vi "MGI Approximately Equal.vi"(1 "Numeric 2":dbl format="%.2f", 2 "Numeric 1":dbl format="%.2f") -> (0 "approx = ?":bool)   [LabVIEW 2020]
doc: "Check that two floats are within 1% of each other. If either number is zero, then check that they are within Machine Epsilon of each other.\n\nAuthored by David A. Moore\nsupport@mooregoodideas.com\nwww.mooregoodideas.com\n\nCopyright (c) 2010, Moore Good Ideas, Inc.\n\nAll rights reserved.\n\nRedistribution and use in source and binary forms, with or without modification, are permitted provided that the following conditions are met:\n\n * Redistributions of source code must retain the above copyright notice, this list of conditions and the following disclaimer.\n * Redistributions in binary form must reproduce the above copyright notice, this list of conditions and the following disclaimer in the documentation and/or other materials provided with the distribution.\n * Neither the name of Moore Good Ideas, Inc. nor the names of its contributors may be used to endorse or promote products derived from this software without specific prior written permission.\n\nTHIS SOFTWARE IS PROVIDED BY THE COPYRIGHT HOLDERS AND CONTRIBUTORS \"AS IS\" AND ANY EXPRESS OR IMPLIED WARRANTIES, INCLUDING, BUT NOT LIMITED TO, THE IMPLIED WARRANTIES OF MERCHANTABILITY AND FITNESS FOR A PARTICULAR PURPOSE ARE DISCLAIMED. IN NO EVENT SHALL THE COPYRIGHT OWNER OR CONTRIBUTORS BE LIABLE FOR ANY DIRECT, INDIRECT, INCIDENTAL, SPECIAL, EXEMPLARY, OR CONSEQUENTIAL DAMAGES (INCLUDING, BUT NOT LIMITED TO, PROCUREMENT OF SUBSTITUTE GOODS OR SERVICES; LOSS OF USE, DATA, OR PROFITS; OR BUSINESS INTERRUPTION) HOWEVER CAUSED AND ON ANY THEORY OF LIABILITY, WHETHER IN CONTRACT, STRICT LIABILITY, OR TORT (INCLUDING NEGLIGENCE OR OTHERWISE) ARISING IN ANY WAY OUT OF THE USE OF THIS SOFTWARE, EVEN IF ADVISED OF THE POSSIBILITY OF SUCH DAMAGE."
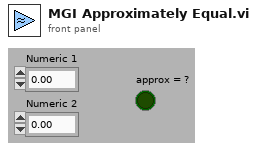
[diagram p1: front panel]
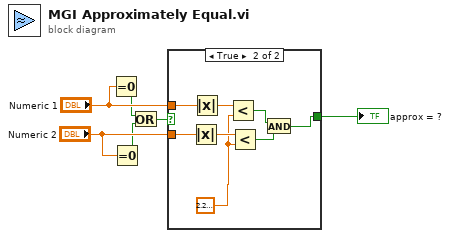
[diagram p0: block diagram]
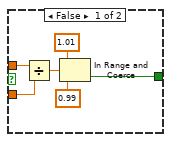
[diagram p2: hidden frame]
diagram:
  n1 = Equal To 0?(x="Numeric 1") -> (x = 0?=w2:bool)
  n2 = Equal To 0?(x="Numeric 2") -> (x = 0?=w3:bool)
  n3 = Or(x=w2, y=w3) -> (x .or. y?=w1:bool)
  n4 = case shown="True" w1 {
    tunnel: [w9 w14] -> w6
    tunnel: "Numeric 2" -> [w8 w19]
    tunnel: "Numeric 1" -> [w7 w20]
    frame False {
      n5 = Divide(x=w7, y=w8) -> (x/y=w12:dbl)
      n6 = In Range and Coerce(upper limit=1.01, x=w12, lower limit=0.99) -> (In Range?=w9:bool)  [unwired: 1 out]
    }
    frame True {
      w13 = 2.220446049250313e-16
      n7 = Absolute Value(x=w19) -> (abs(x)=w17:dbl)
      n8 = Absolute Value(x=w20) -> (abs(x)=w18:dbl)
      n9 = Less?(x=w18, y=w13) -> (x < y?=w16:bool)
      n10 = Less?(x=w17, y=w13) -> (x < y?=w15:bool)
      n11 = And(x=w16, y=w15) -> (x .and. y?=w14:bool)
    }
  }
  "approx = ?" <- w6
